vi "Configure Standard Waveform(Noise).vi"(0 "VISA resource name":refnum<visa-resource-name>, 5 "Output Channel (1: Channel 1)":i32(ring)=1 items=["Channel 1"=1, "Channel 2"=2], 7 "Amplitude (5)":dbl=5.0, 9 "Amplitude Unit (0: Vpp)":i32(ring) items=["Vpp", "Vrms", "dBm"], 11 "error in (no error)":errorcluster, 12 "Offset (0)":dbl) -> (4 "VISA resource name out":refnum<visa-resource-name>, 15 "error out":errorcluster)   [LabVIEW 2012, in "RIGOL DG4000 Series.lvlib"]
doc: "Outputs a noise with specified amplitude and DC offset."
uses:
  <instrlib>/RIGOL DG4000 Series/RIGOL DG4000 Series.lvlib
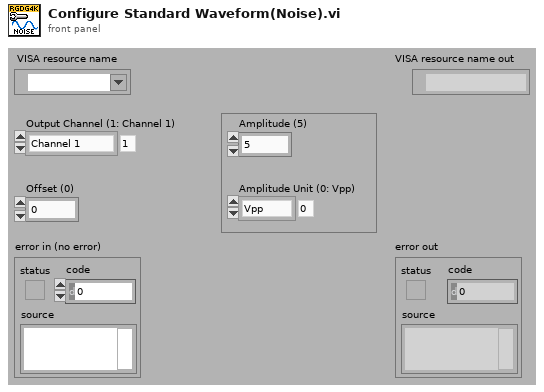
[diagram p1: front panel]
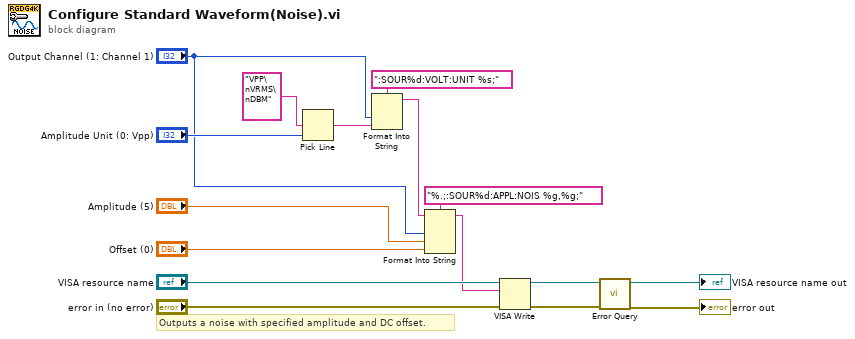
[diagram p0: block diagram]
diagram:
  # "Outputs a noise with specified amplitude and DC offset."
  n1 = Pick Line(multi-line string="VPP\nVRMS\nDBM", line index="Amplitude Unit (0: Vpp)") -> (output string=w10:string)  [unwired: 1 out]
  n2 = Format Into String(format string=":SOUR%d:VOLT:UNIT %s;", "Output Channel (1: Channel 1)", w10) -> (resulting string=w2:string)  [unwired: 2 in, 1 out]
  n3 = Format Into String(format string="%.;:SOUR%d:APPL:NOIS %g,%g;", initial string=w2, "Output Channel (1: Channel 1)", "Amplitude (5)", "Offset (0)") -> (resulting string=w1:string)  [unwired: 1 in, 1 out]
  n4 = VISA Write(VISA resource name="VISA resource name", write buffer=w1, error in (no error)="error in (no error)") -> (VISA resource name out=w7:refnum<visa-resource-name>, error out=w6:errorcluster)  [unwired: 1 out]
  n5 = call <instrlib>:"Error Query.vi"("error in (no error)"=w6, "VISA resource name"=w7) -> ("error out"=→"error out":errorcluster, "VISA resource name out"=→"VISA resource name out":refnum<visa-resource-name>)  [unwired: 8 out]
